vi "Untitled 4.vi"() -> ()   [LabVIEW 2012]
uses:
  <vilib>/userdefined/High Color/IMAQdx.ctl
  <vilib>/vision/driver/NI_Vision_Acquisition_Software.lvlib
panel:
  out "Image":T1(plugin-control)
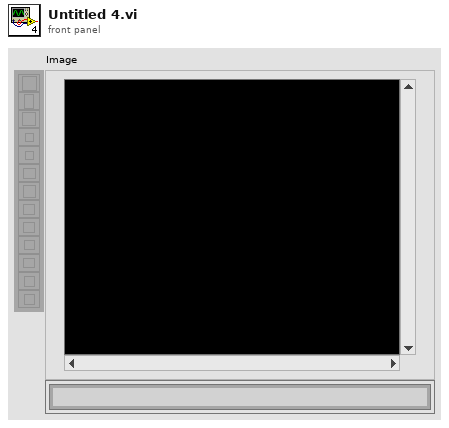
[diagram p1: front panel]
types:
  T1 = typedef "IMAQ Image.ctl" = refnum<image>
  T2 = typedef "IMAQdx.ctl" = refnum<k21>
  T3 = typedef "Image Type" = u32
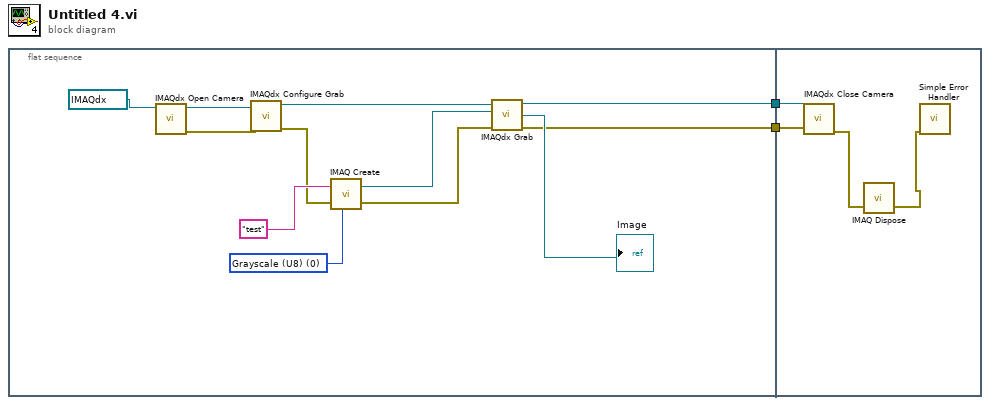
[diagram p0: block diagram]
diagram:
  n1 = flat-sequence {
    tunnel: [w12] -> w2
    tunnel: [w11] -> w1
    tunnel: w2 -> [w16]
    tunnel: w1 -> [w15]
    frame #0 {
      w6 = T3 0 items=["Grayscale (U8)", "Grayscale (I16)", "Grayscale (SGL)", "Complex (CSG)", "RGB (U32)", "HSL (U32)", "RGB (U64)", "Grayscale (U16)"] ("Image Type")
      n2 = call <vilib>:"IMAQdx Open Camera.vi"("Session In"=T2 "cam0") -> ("error out"=w8:errorcluster, "Session Out"=w10:T2)  [unwired: 9 in]
      n3 = call <vilib>:"IMAQdx Configure Grab.vi"("error in"=w8, "Session In"=w10) -> ("error out"=w4:errorcluster, "Session Out"=w9:T2)  [unwired: 8 in]
      n4 = call "IMAQ Create"("Image Name"="test", "Image Type"=w6, "error in (no error)"=w4) -> ("New Image"=w5:T1, "error out"=w3:errorcluster)  [unwired: 1 in, 1 out]
      n5 = call <vilib>:"IMAQdx Grab.vi"("error in"=w3, "Image In"=w5, "Session In"=w9) -> ("error out"=w11:errorcluster, "Image Out"=→"Image":T1, "Session Out"=w12:T2)  [unwired: 5 in, 1 out]
    }
    frame #1 {
      n6 = call <vilib>:"IMAQdx Close Camera.vi"("error in"=w15, "Session In"=w16) -> ("error out"=w18:errorcluster)  [unwired: 9 in]
      n7 = call "IMAQ Dispose"("error in (no error)"=w18) -> ("error out"=w17:errorcluster)  [unwired: 2 in, 3 out]
      n8 = call <vilib>:"Simple Error Handler.vi"("error in (no error)"=w17) -> ()  [unwired: 1 in, 8 out]
    }
  }
